vi "map.vi"(0 "WebBrowser":refnum<k7>(container), 1 "纬度":ext=113.69712352752688, 2 "经度":ext=34.79248399030799) -> ()   [LabVIEW 2012]
panel:
  in  "HTML":string="<!DOCTYPE html PUBLIC \"-//W3C//DTD XHTML 1.0 Transitional//EN\" \"http://www.w3.org/TR/xhtml1/DTD/xhtml1-transitional.dtd\">\n<html>\n   <head>\n      <title></title>\n      <meta http-equiv=\"Content-Type\" content=\"text/html; charset=utf-8\">\n      <script type=\"text/javascript\" src=\"http://dev.ditu.live.com/mapcontrol/mapcontrol.ashx?v=6.1\"></script>\n      <script type=\"text/javascript\">\n         var map = null;\n                   \n         function GetMap()\n         {\n            map = new VEMap('myMap');\n            map.LoadMap();\n            map.SetZoomLevel(14);\n            var latLon=new VELatLong(经度的位置,纬度的位置);  \n            //设置地图中心点  \n            map.SetCenter(latLon);  \n         }\n        \n      </script>\n   </head>\n   <body onload=\"GetMap();\">\n      <div id='myMap' style=\"position:relative; width:800px; height:600px;\"></div>\n       <br/>\n   </body>\n</html>"
  out "innerHTML":string
  out "Container":bool
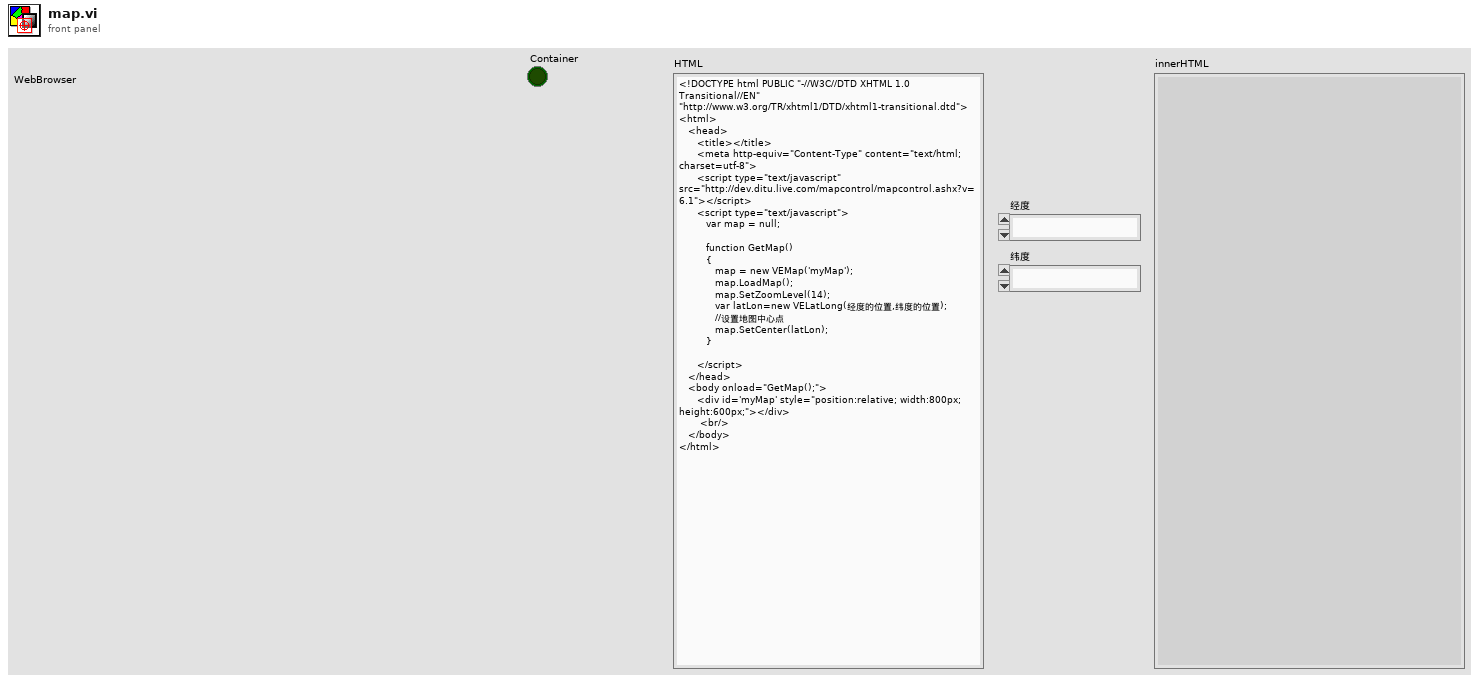
[diagram p1: front panel]
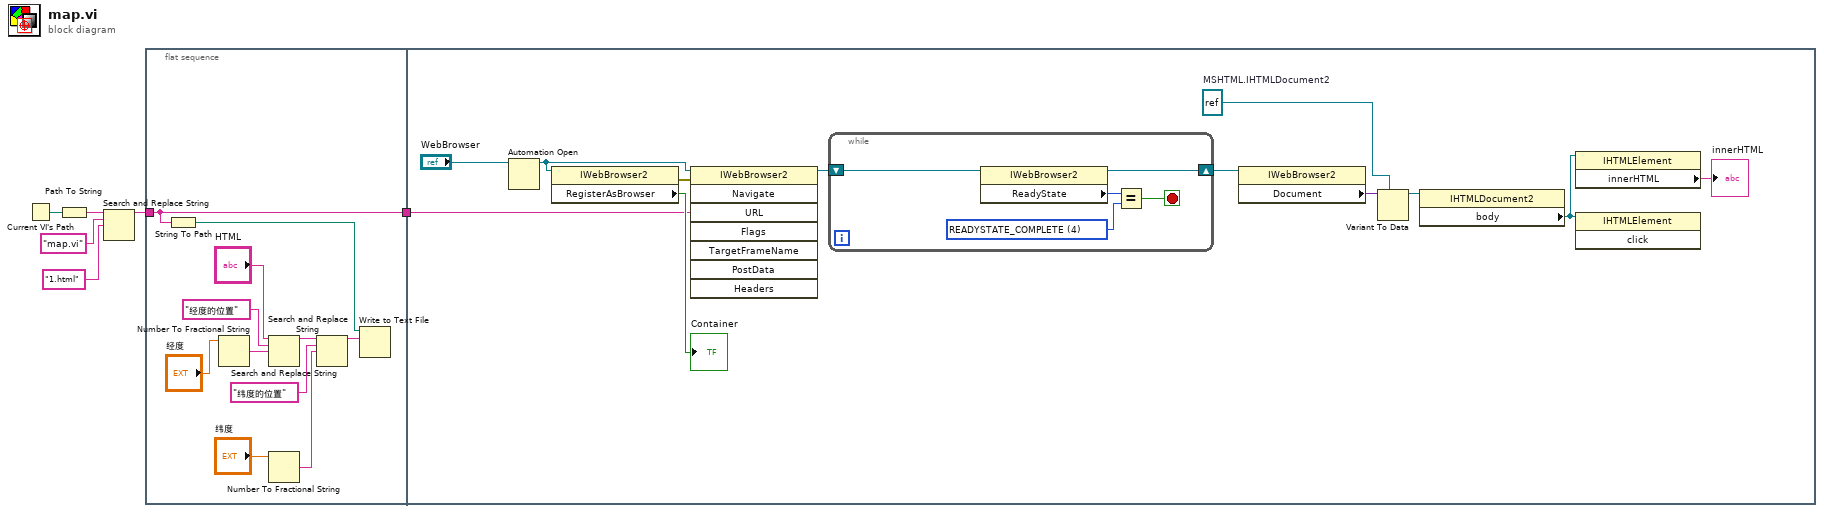
[diagram p0: block diagram]
diagram:
  n1 = Current VI's Path() -> (path=w5:path)
  n2 = Path To String(path=w5) -> (string=w4:string)
  n3 = Search and Replace String(input string=w4, search string="map.vi" ("URL"), replace string="1.html" ("URL")) -> (result string=w1:string)  [unwired: 5 in, 3 out]
  n4 = flat-sequence {
    tunnel: [w7] -> w6
    tunnel: w1 -> [w7]
    tunnel: w6 -> [w18]
    frame #0 {
      n5 = String To Path(string=w7) -> (path=w8:path)
      n6 = Number To Fractional String(number="经度") -> (F-format string=w12:string)  [unwired: 3 in]
      n7 = Search and Replace String(input string="HTML", search string="经度的位置" ("URL"), replace string=w12) -> (result string=w13:string)  [unwired: 5 in, 3 out]
      n8 = Number To Fractional String(number="纬度") -> (F-format string=w16:string)  [unwired: 3 in]
      n9 = Search and Replace String(input string=w13, search string="纬度的位置" ("URL"), replace string=w16) -> (result string=w17:string)  [unwired: 5 in, 3 out]
      n10 = Write to Text File(file (use dialog)=w8, text=w17) -> ()  [unwired: 2 in, 3 out]
    }
    frame #1 {
      w27 = refnum<k7> refnum  # MSHTML.IHTMLDocument2
      n11 = Automation Open(Automation Refnum="WebBrowser") -> (Automation Refnum=w23:refnum<k7>)  [unwired: 3 in, 1 out]
      n12 = property class="IWebBrowser2"(reference=w23) -> (error out=w24:errorcluster, "RegisterAsBrowser"=→"Container":bool)  [unwired: 1 in, 1 out]
      n13 = invoke class="IWebBrowser2" method="Navigate"(reference=w23, error in=w24, "URL"=w18) -> (reference out=w21:refnum<k7>)  [unwired: 5 in, 7 out]
      n14 = while {
        shift-right: [w31] -> w20
        shift-left: w21 -> [w30]
        stop <- w32 stop-if-true
        w33 = 4 items=["READYSTATE_UNINITIALIZED", "READYSTATE_LOADING", "READYSTATE_LOADED", "READYSTATE_INTERACTIVE", "READYSTATE_COMPLETE"] ("ReadyState")
        n15 = property class="IWebBrowser2"(reference=w30) -> (reference out=w31:refnum<k7>, "ReadyState"=w34:i32)  [unwired: 1 in, 1 out]
        n16 = Equal?(x=w34, y=w33) -> (x = y?=w32:bool)
      }
      n17 = property class="IWebBrowser2"(reference=w20) -> ("Document"=w26:variant)  [unwired: 1 in, 2 out]
      n18 = Variant To Data(type=w27, Variant=w26) -> (data=w28:refnum<k7>)  [unwired: 1 in, 1 out]
      n19 = property class="IHTMLDocument2"(reference=w28) -> ("body"=w29:refnum<k7>)  [unwired: 1 in, 2 out]
      n20 = property class="IHTMLElement"(reference=w29) -> ("innerHTML"=→"innerHTML":string)  [unwired: 1 in, 2 out]
      n21 = invoke class="IHTMLElement" method="click"(reference=w29) -> ()  [unwired: 2 in, 3 out]
    }
  }
